vi "Goniometer.vi"() -> ()   [LabVIEW 2024]
uses:
  F:/Desktop/Goniometer_Labview/ThorLabs.MotionControl.KCube.DCServoCLI.dll
  ThorLabs.MotionControl.KCube.DCServoCLI.dll
  <vilib>/Utility/file.llb/Write Delimited Spreadsheet (DBL).vi
  F:/Desktop/Goniometer_Labview/Thorlabs.MotionControl.Controls.dll
  Thorlabs.MotionControl.Controls.dll
panel:
  out "transposed array":dbl[][](array[numeric])
  in  "file path (dialog if empty)":path
  out "이동거리":dbl[](array[numeric])
  out "Waveform Chart":dbl[](graph)
  out "XY Graph":cluster{dbl[], dbl[]}(graph)
  out "측정값":dbl[](array[numeric])
  out "error out":errorcluster {"code" format="%.0x"}
  in  "direction":i32(ring)=2 items=["Forward"=1, "Backward"=2]
  in  "목표각":dbl
  in  "간격각도":dbl
  in  "Mode":u16(ring) items=["Current", "Power"]
  out "Current":dbl
  in  "Wavelength (0.0)":dbl=1064.0
  out "Power":dbl
  in  "Serial Number":string
  in  "KCubeDCServoControl":refnum<k24>(container)
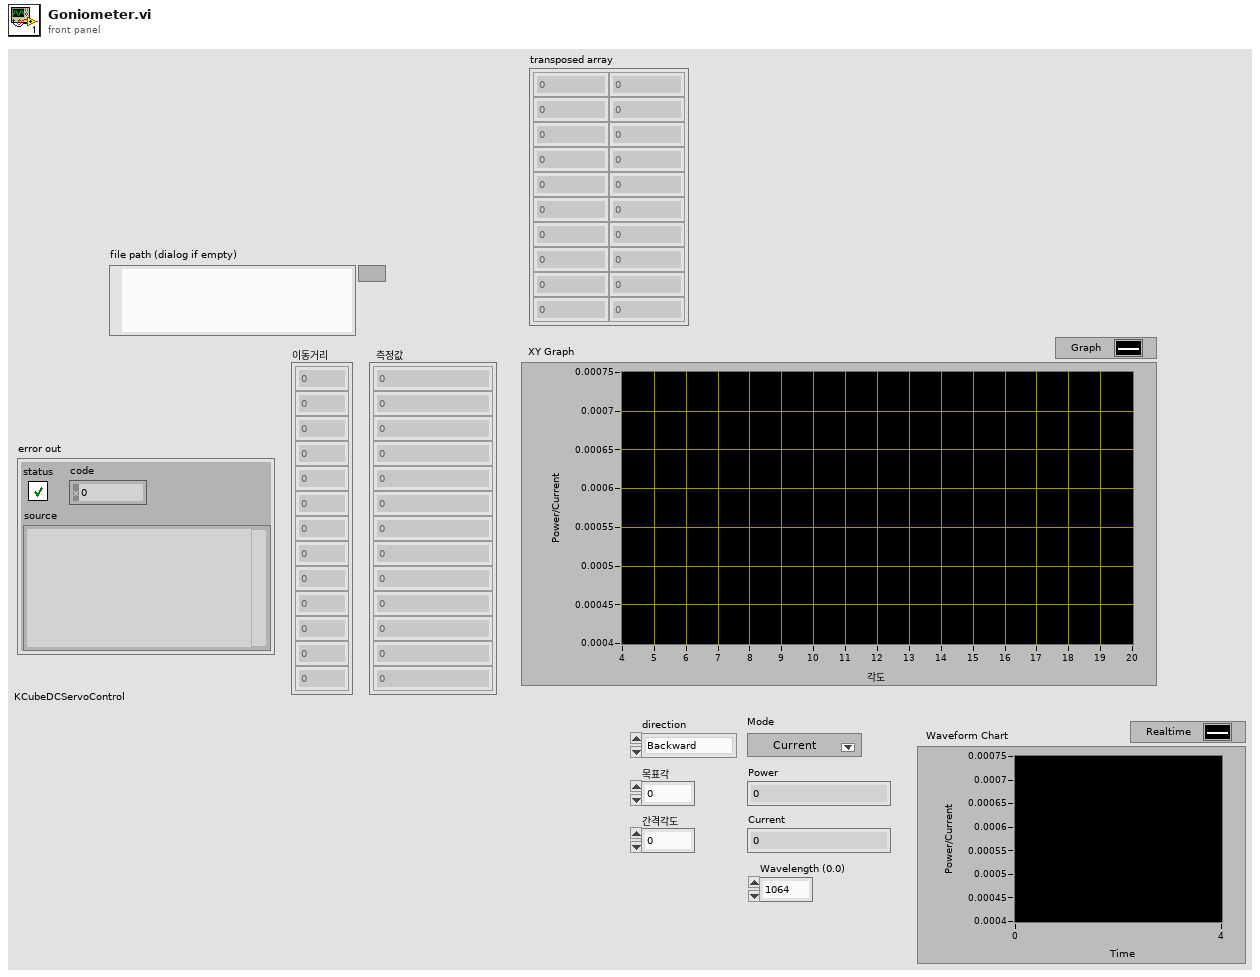
[diagram p1: front panel]
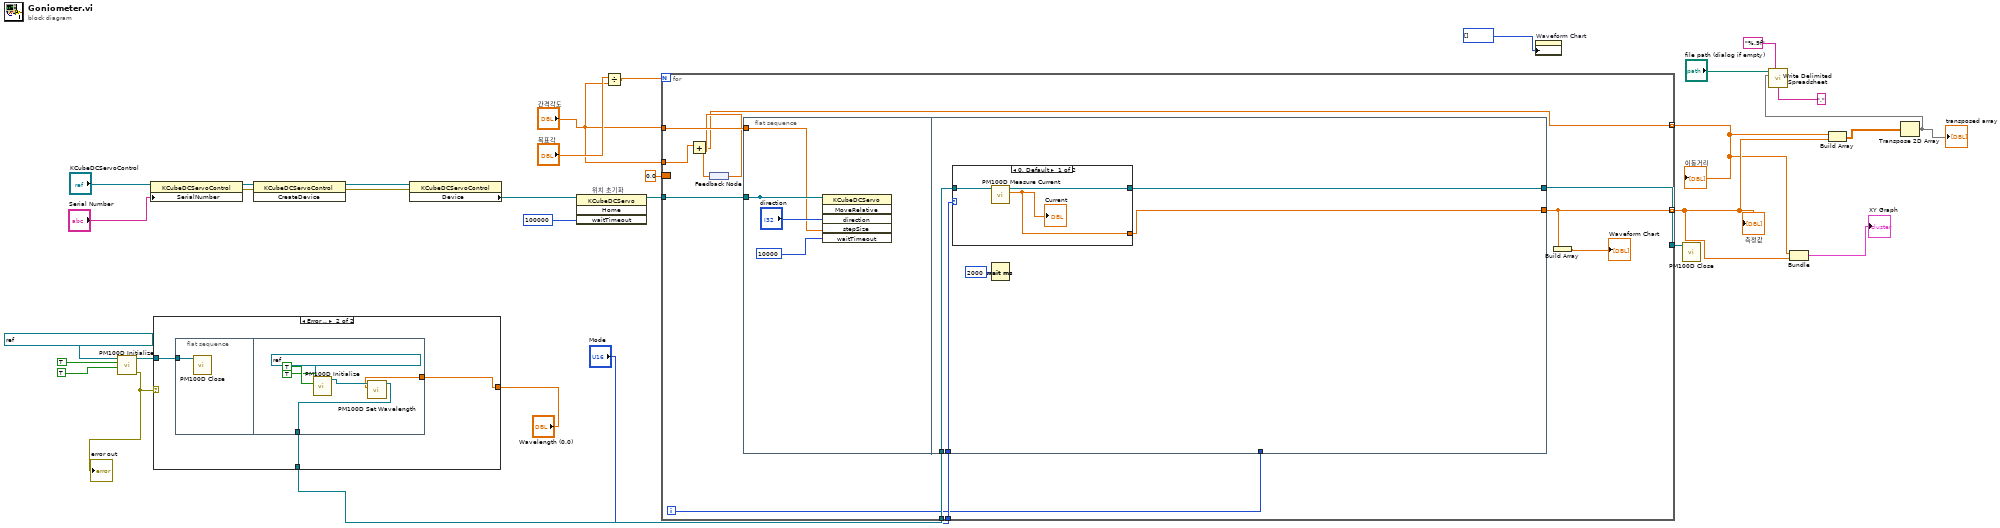
[diagram p0: block diagram]
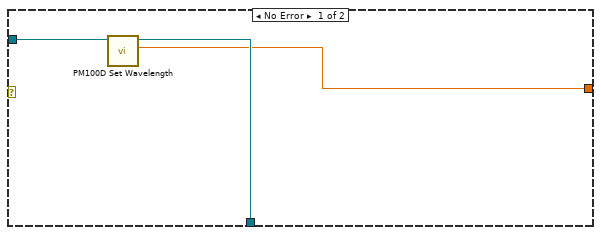
[diagram p2: hidden frame]
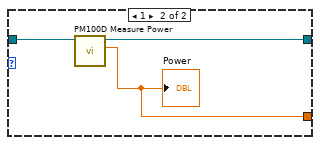
[diagram p3: hidden frame]
diagram:
  n1 = call <instrlib>:"PM100D Initialize.vi"("Reset Device (Reset Device)"=TRUE, "ID Query (Do Query)"=TRUE, "resource name"=refnum<visa-resource-name> "USB0::0x1313::0x8078::P0008024::INSTR") -> ("error out"=w13:errorcluster, "instrument handle out"=w22:refnum<visa-resource-name>)  [unwired: 7 in]
  "error out" <- w13
  n2 = property class="KCubeDCServoControl"(reference="KCubeDCServoControl", "SerialNumber"="Serial Number") -> (reference out=w27:refnum<k24>, error out=w30:errorcluster)  [unwired: 1 in]
  n3 = case shown="Error .." w13 {
    tunnel: w22 -> [w34 w37]
    tunnel: [w33 w36] -> w19
    tunnel: "Wavelength (0.0)" -> [w32 w35]
    frame No Error {
      n4 = call <instrlib>:"PM100D Set Wavelength.vi"("Wavelength (0.0)"=w32, "instrument handle"=w34) -> ("instrument handle out"=w33:refnum<visa-resource-name>)  [unwired: 8 in, 1 out]
    }
    frame Error {
      n5 = flat-sequence {
        tunnel: w37 -> [w38]
        tunnel: [w40] -> w36
        tunnel: w35 -> [w39]
        frame #0 {
          n6 = call <instrlib>:"PM100D Close.vi"("instrument handle"=w38) -> ()  [unwired: 10 in, 1 out]
        }
        frame #1 {
          n7 = call <instrlib>:"PM100D Initialize.vi"("Reset Device (Reset Device)"=TRUE, "ID Query (Do Query)"=TRUE, "resource name"=refnum<visa-resource-name> "USB0::0x1313::0x8078::P0008024::INSTR") -> ("instrument handle out"=w41:refnum<visa-resource-name>)  [unwired: 7 in, 1 out]
          n8 = call <instrlib>:"PM100D Set Wavelength.vi"("Wavelength (0.0)"=w39, "instrument handle"=w41) -> ("instrument handle out"=w40:refnum<visa-resource-name>)  [unwired: 8 in, 1 out]
        }
      }
    }
  }
  n9 = invoke class="KCubeDCServoControl" method="CreateDevice"(reference=w27, error in=w30) -> (reference out=w28:refnum<k24>, error out=w31:errorcluster)  [unwired: 1 in, 1 out]
  n10 = property class="KCubeDCServoControl"(reference=w28, error in=w31) -> ("Device"=w16:refnum<k24>)  [unwired: 2 out]
  n11 = invoke on="위치 초기화" class="KCubeDCServo" method="Home"(reference=w16, "waitTimeout"=100000) -> (reference out=w15:refnum<k24>)  [unwired: 2 in, 3 out]
  n12 = Divide(x="목표각", y="간격각도") -> (x/y=w21:dbl)
  n13 = for {
    N: w21 -> [_]
    tunnel: w15 -> [w55]
    tunnel: "Mode" -> [w54]
    tunnel: "간격각도" -> [w53]
    tunnel: w19 -> [w52]
    tunnel: [w51] -> w18
    tunnel: "간격각도" -> [w49]
    tunnel: [w47] -> w6 mode=indexing
    tunnel: [w45] -> w3 mode=indexing
    border: 0.0 -> [_]
    i -> [w50]
    n14 = feedback #1() -> (w48:dbl)
    n15 = Add(x=w49, y=w48) -> (x+y=w45:dbl)
    n16 = feedback-in #1(w45) -> ()
    n17 = flat-sequence {
      tunnel: w53 -> [w56]
      tunnel: w55 -> [w59]
      tunnel: [w59] -> _
      tunnel: w54 -> [w64]
      tunnel: w52 -> [w63]
      tunnel: [w62] -> w51
      tunnel: w50 -> [_]
      tunnel: [w60] -> w47
      frame #0 {
        n18 = invoke class="KCubeDCServo" method="MoveRelative"(reference=w59, "direction"="direction", "stepSize"=w56, "waitTimeout"=10000) -> ()  [unwired: 2 in, 6 out]
      }
      frame #1 {
        n19 = case shown="0, Default" w64 {
          tunnel: w63 -> [w66 w70]
          tunnel: [w67 w69] -> w62
          tunnel: [w65 w68] -> w60
          frame 0, Default {
            n20 = call <instrlib>:"PM100D Measure Current.vi"("instrument handle"=w66) -> ("Current"=w65:dbl, "instrument handle out"=w67:refnum<visa-resource-name>)  [unwired: 8 in, 1 out]
            "Current" <- w65
          }
          frame 1 {
            n21 = call <instrlib>:"PM100D Measure Power.vi"("instrument handle"=w70) -> ("Power"=w68:dbl, "instrument handle out"=w69:refnum<visa-resource-name>)  [unwired: 8 in, 1 out]
            "Power" <- w68
          }
        }
        n22 = Wait (ms)(milliseconds to wait=u32 2000) -> ()  [unwired: 1 out]
      }
    }
    n23 = Build Array(w47) -> (→"Waveform Chart":dbl[])
  }
  "측정값" <- w6
  "이동거리" <- w3
  n24 = property on="Waveform Chart" class="WFChart (strict)"("History Data"=i32[] []) -> ()  [unwired: 2 in, 2 out]
  n25 = call <instrlib>:"PM100D Close.vi"("instrument handle"=w18) -> ()  [unwired: 10 in, 1 out]
  n26 = Bundle(w3, w6) -> (→"XY Graph":cluster{dbl[], dbl[]})  [unwired: 1 in]
  n27 = Build Array(w3, w6) -> (w5:dbl[][])
  n28 = Transpose 2D Array(2D array=w5) -> (transposed array=w4:dbl[][])
  "transposed array" <- w4
  n29 = call-poly <vilib>:"Write Delimited Spreadsheet.vi"("file path (dialog if empty)"="file path (dialog if empty)", "format (%.3f)"="%.9f", "2D data"=w4, "delimiter (\\t)"="," ("delimiter (\\t)")) -> ()  [unwired: 10 in, 2 out]
